vi "Start Flow.vi"   [LabVIEW 2015, in "Global FIA milliGAT.lvlib"]
uses:
  Global FIA milliGAT.lvlib
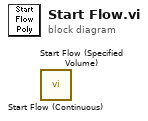
[diagram p0: block diagram]
diagram:
  n1 = call "Start Flow (Continuous).vi"() -> ()  [unwired: 10 in, 2 out]
  n2 = call "Start Flow (Specified Volume).vi"() -> ()  [unwired: 10 in, 2 out]
